vi "Write _To_CSV_File.vi"(0 "Refnum In":refnum<file>, 1 "String Array 1":string[](array[string]), 2 "String Array 2":string[](array[string]), 3 "String Array 3":string[](array[string]), 5 "Error In":errorcluster) -> (14 "Refnum Out":refnum<file>, 15 "File Path":path, 19 "Error Out":errorcluster)   [LabVIEW 2021]
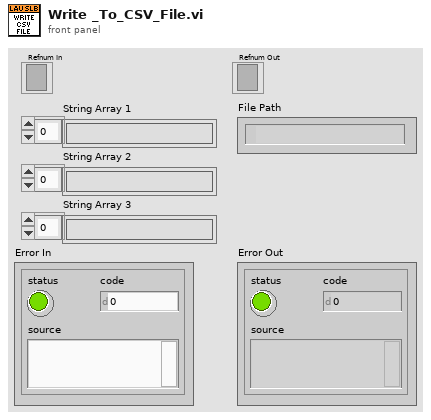
[diagram p1: front panel]
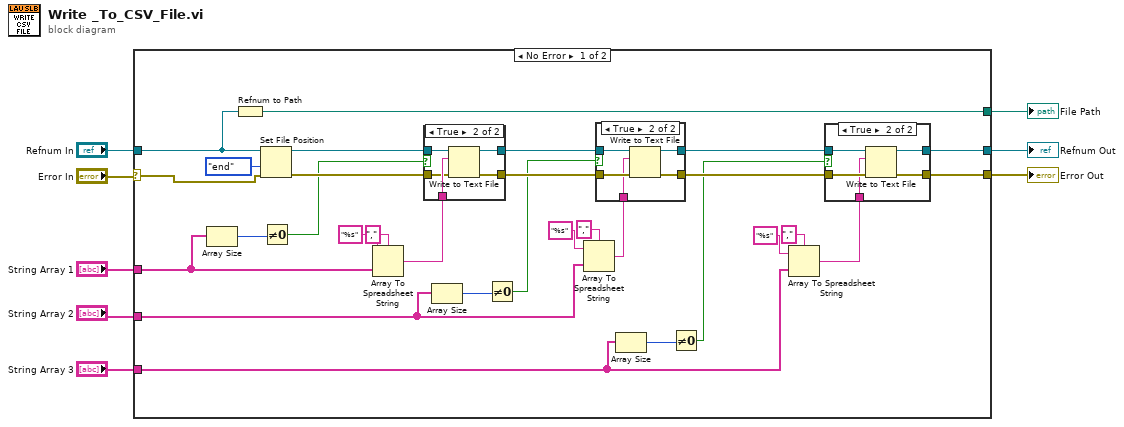
[diagram p0: block diagram]
diagram:
  n1 = case shown="No Error" "Error In" {
    selector: "Error In" -> [w35 w60]
    tunnel: [w19 _] -> w7
    tunnel: [w21 w60] -> w6
    tunnel: [w26 _] -> w5
    tunnel: "Refnum In" -> [w25 _]
    tunnel: "String Array 1" -> [w17 _]
    tunnel: "String Array 2" -> [w13 _]
    tunnel: "String Array 3" -> [w10 _]
    frame No Error {
      n2 = Array Size(array=w17) -> (size(s)=w16:i32)
      n3 = Refnum to Path(1:w25) -> (0:w26:path)
      n4 = Set File Position(refnum=w25, from (0:start)=enum16{"start", "end", "current"}."end", error in=w35) -> (refnum out=w32:refnum<file>, error out=w34:errorcluster)  [unwired: 1 in]
      n5 = Not Equal To 0?(x=w16) -> (x != 0?=w15:bool)
      n6 = Array To Spreadsheet String(delimiter (Tab)=",", array=w17, 3:"%s" ("format string")) -> (spreadsheet string=w36:string)
      n7 = case shown="True" w15 {
        tunnel: w36 -> [_ w59]
        tunnel: w34 -> [w54 w58]
        tunnel: w32 -> [w53 w57]
        tunnel: [w54 w56] -> w31
        tunnel: [w53 w55] -> w27
        frame False {
        }
        frame True {
          n8 = Write to Text File(file (use dialog)=w57, text=w59, error in=w58) -> (refnum out=w55:refnum<file>, error out=w56:errorcluster)  [unwired: 1 in, 1 out]
        }
      }
      n9 = Array Size(array=w13) -> (size(s)=w14:i32)
      n10 = Not Equal To 0?(x=w14) -> (x != 0?=w12:bool)
      n11 = Array To Spreadsheet String(delimiter (Tab)=",", array=w13, 3:"%s" ("format string")) -> (spreadsheet string=w28:string)
      n12 = case shown="True" w12 {
        tunnel: w31 -> [w46 w52]
        tunnel: w28 -> [_ w51]
        tunnel: w27 -> [w47 w50]
        tunnel: [w46 w49] -> w22
        tunnel: [w47 w48] -> w20
        frame False {
        }
        frame True {
          n13 = Write to Text File(file (use dialog)=w50, text=w51, error in=w52) -> (refnum out=w48:refnum<file>, error out=w49:errorcluster)  [unwired: 1 in, 1 out]
        }
      }
      n14 = Array Size(array=w10) -> (size(s)=w11:i32)
      n15 = Not Equal To 0?(x=w11) -> (x != 0?=w9:bool)
      n16 = Array To Spreadsheet String(delimiter (Tab)=",", array=w10, 3:"%s" ("format string")) -> (spreadsheet string=w18:string)
      n17 = case shown="True" w9 {
        tunnel: w22 -> [w39 w45]
        tunnel: [w39 w44] -> w21
        tunnel: w20 -> [w40 w43]
        tunnel: [w40 w42] -> w19
        tunnel: w18 -> [_ w41]
        frame False {
        }
        frame True {
          n18 = Write to Text File(file (use dialog)=w43, text=w41, error in=w45) -> (refnum out=w42:refnum<file>, error out=w44:errorcluster)  [unwired: 1 in, 1 out]
        }
      }
    }
    frame Error {
    }
  }
  "Error Out" <- w6
  "Refnum Out" <- w7
  "File Path" <- w5
